vi "Get iterations.vi"() -> (0 "Screen update":i32, 1 "Momentum":dbl=1.0 format="%.2f", 2 "RMS to quit":dbl=2.0 format="%.2f", 3 "Total iterations":i32=1000, 4 "Continue? (T=yes)":bool=TRUE)   [LabVIEW 2010]
panel:
  in  "Momentum":dbl=0.8 format="%.2f"
  in  "RMS error to quit (%)":dbl=1.0 format="%.2f"
  in  "Screen update":i32=5
  in  "Total number of iterations":i32=10000
  in  "Exit":bool
  in  "OK":bool
  # "Set Iterations...\n(you can change any of these settings later)"
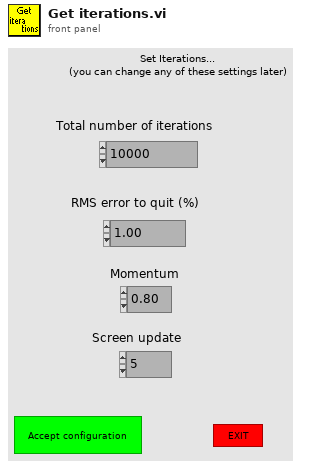
[diagram p1: front panel]
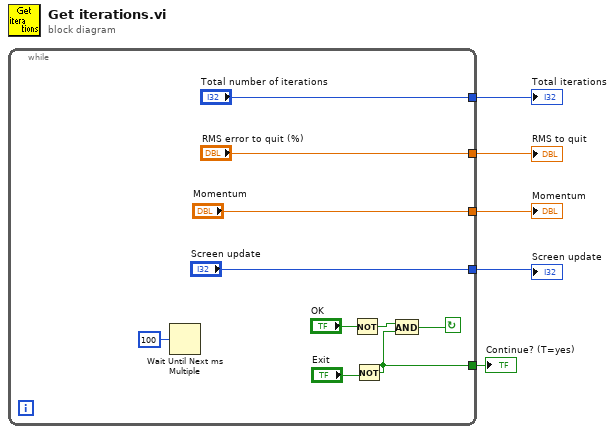
[diagram p0: block diagram]
diagram:
  n1 = while {
    tunnel: ["Screen update"] -> w1
    tunnel: ["Momentum"] -> w2
    tunnel: ["RMS error to quit (%)"] -> w3
    tunnel: ["Total number of iterations"] -> w4
    tunnel: [w11] -> w5
    stop <- w12 continue-if-true
    n2 = Wait Until Next ms Multiple(millisecond multiple=u32 100) -> ()  [unwired: 1 out]
    n3 = Not(x="OK") -> (.not. x?=w14:bool)
    n4 = Not(x="Exit") -> (.not. x?=w11:bool)
    n5 = And(x=w14, y=w11) -> (x .and. y?=w12:bool)
  }
  "Continue? (T=yes)" <- w5
  "RMS to quit" <- w3
  "Momentum" <- w2
  "Screen update" <- w1
  "Total iterations" <- w4
